vi "Calculate Stim-Recovery Amplitude.vi"(8 "error in":errorcluster, 11 "waveform":waveform(dbl)={"t0"=timestamp(3473168073.631 s since 1904-01-01), "dt"=1e-08, "Y"=[], "attributes"=variant("Average Size"=variant(dbl 15.0), "NSamp"=variant(dbl 400000.0), "Resistance (ohms)"=variant(dbl 500.0), "Samp Freq (MHz)"=variant(dbl 100.0), "dt (us)"=variant(dbl 0.01))}) -> (0 "error out":errorcluster, 1 "Recvy Amp (V)":dbl=nan format="%.4p", 2 "Stim Amp (V)":dbl=nan format="%.4p", 3 "waveform out":waveform(dbl)={"t0"=timestamp(3472747248.0780005 s since 1904-01-01), "dt"=nan, "Y"=[]})   [LabVIEW 2010]
doc: "This function calculates minimum and maximum pulse levels, then determines which levels are the stimulus and recovery amplitudes. Amplitudes are stored as waveform attributes in double precision floating point format.\n\nIf there is an external error or calculation error, then \"Stim Amp (V)\" and \"Recvy Amp (V)\" are set to NaN. Any calculation errors are cleared to allow further processing to continue.\n\nThese measurements are consistent with the IEEE Standard 181-2003, Standard on Transitions, Pulses, and Related Waveforms."
uses:
  <vilib>/measure/mascope.llb/Amplitude and Levels 1 chan.vi
  <vilib>/measure/NI_MAPro.lvlib
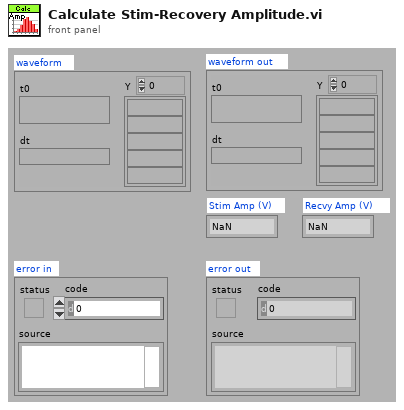
[diagram p1: front panel]
types:
  T1 = cluster{"method":enum32{"histogram", "peak", "auto select"}, "histogram size":i32, "histogram method":enum16{"mode"}, "reserved":dbl}
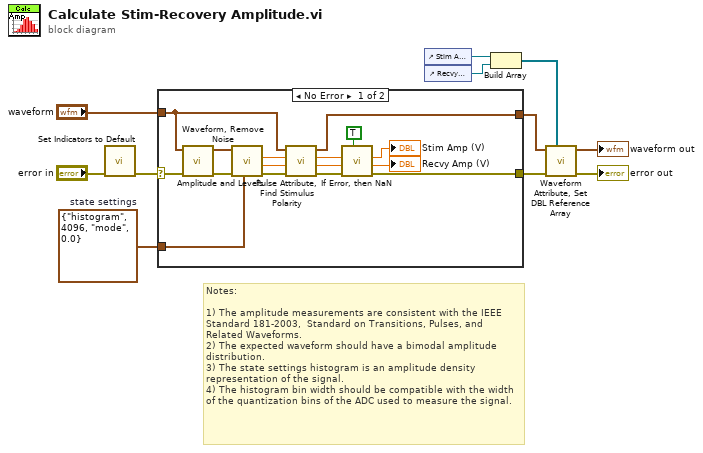
[diagram p0: block diagram]
diagram:
  w7 = T1 {"method"=enum."histogram", "histogram size"=4096, "histogram method"=enum."mode", "reserved"=0.0}  # state settings
  # "Notes:\n\n1) The amplitude measurements are consistent with the IEEE Standard 181-2003,  Standard on Transitions, Pulses, and Related Waveforms.\n2) The expected waveform should have a bimodal amplitude distribution.\n3) The state settings histogram is an amplitude density representation of the signal.\n4) The histogram bin width should be compatible with the width of the quantization bins of the ADC used to measure the signal."
  n1 = call "Set Indicators to Default.vi"("error in"="error in") -> ("error out"=w1:errorcluster)  [unwired: 6 in]
  n2 = case shown="No Error" w1 {
    selector: w1 -> [w15 w29]
    tunnel: "waveform" -> [w13 w28]
    tunnel: [w21 w29] -> w11
    tunnel: w7 -> [w25 _]
    tunnel: [w22 w28] -> w3
    frame No Error {
      n3 = call "Waveform, Remove Noise.vi"("error in"=w15, "waveform"=w13) -> ("error out"=w14:errorcluster, "waveform out"=w12:waveform(dbl))  [unwired: 7 in]
      n4 = call-poly <vilib>:"Amplitude and Levels.vi"("state settings"=w25, "error in (no error)"=w14, "signal in"=w12) -> ("error out"=w27:errorcluster, "low state level"=w23:dbl, "high state level"=w24:dbl)  [unwired: 5 in, 1 out]
      n5 = call "Pulse Attribute, Find Stimulus Polarity.vi"("error in"=w27, "amp min"=w23, "amp max"=w24, "waveform"=w13) -> ("error out"=w26:errorcluster, "Recvy Amp"=w20:dbl, "Stim Amp"=w19:dbl, "waveform out"=w22:waveform(dbl))  [unwired: 4 in]
      n6 = call "If Error, then NaN.vi"("clear error (F)"=TRUE, "error in (T)"=w26, "value3"=w20, "value2"=w19) -> ("error out"=w21:errorcluster, "value out3"=→"Recvy Amp (V)":dbl, "value out2"=→"Stim Amp (V)":dbl)  [unwired: 2 in, 1 out]
    }
    frame Error {
    }
  }
  n7 = control-ref of="Stim Amp (V)"() -> (w5:refnum<vi>)
  n8 = control-ref of="Recvy Amp (V)"() -> (w4:refnum<vi>)
  n9 = Build Array(w5, w4) -> (w6:refnum<vi>[])
  n10 = call "Waveform Attribute, Set DBL Reference Array.vi"("Refnum Array"=w6, "error in"=w11, "waveform"=w3) -> ("error out"=→"error out":errorcluster, "waveform out"=→"waveform out":waveform(dbl))  [unwired: 5 in]
